vi "fgv_params_save-load_manual.vi"(7 "cmd":T8(ring), 8 "error in":errorcluster, 11 "file name":string) -> (0 "error out":errorcluster, 2 "Params_all":T1={"DL950_config"={"Timeout"=10000, "Time Div"=19, "Acq Mode"=0, "Record Len"=5, "Record Num"=0, "Start Point"=0, "End Poin"=60000, "Visa"="TCPIP0::192.168.0.100::inst0::INSTR", "Config Voltage"=[{"Enable"=TRUE, "Ch"=0, "V Div"=12, "Coupling"=1, "Probe"=3, "Act.Items"=FALSE, "items"=[]}, {"Enable"=TRUE, "Ch"=0, "V Div"=12, "Coupling"=1, "Probe"=3, "Act.Items"=FALSE, "items"=[]}], "Trigger on"=FALSE, "Trigger Level"=0.0, "Reset"=FALSE, "Config Temp"=[], "Trig Mode"=1, "Trig Pos"=50.0, "Trigger Slope"=0, "Trigger Source "=1, "Trig Start -5"=-5.0, "End 5"=5.0}, "BP4610 Config"={"VISA"="", "Limit-BP"={"Set"=enum."Current", "Voltage+[V]"=20.0, "Current+[A]"=5.0, "Voltage-[V]"=-20.0, "Current-[A]"=-5.0}, "SET BP"={"Set"=enum."FREQ/WAVE", "Operation mode"=0, "Voltage[Vp-p]"=0.0, "Current[Ap-p]"=0.0, "Voltage[V]"=0.0, "Current[A]"=0.0, "Frequency[Hz]"=1.0, "Waveform"=enum."Sine"}}, "DSP1950 Config"={"Port"="TCPIP0::192.168.0.14::HISLIP0::INSTR", "OVP Level"=0.0, "OCP Level"=0.0, "Current"=0.0, "Voltage"=0.0}, "DMM 2470 Config"={"Source Mode"=enum."Voltage", "Source Limit Level"=0.01, "Source Level"=0.0, "Output_2470"=FALSE}, "cDAQ-9221 Config"={"input terminal"=10083, "minimum value"=-60.0, "maximum value"=60.0, "number of samples"=1000, "rate"=10000.0, "sample mode"=10123, "physical channels"=""}, "cDAQ-9467 Config"="", "cDAQ-9269 AO Config"={"Ch"="cDAQ1Mod1/ao0", "Max V"=5.0, "Min V"=-5.0, " Rate"=1000.0, "N pts"=100, "sample mode"=10178}, "AO_Wave-config"={"offset"=0.0, "Samples"=0, "duty"=0.0, "Rate"=0.0, "wfm"={"Freq"=0.0, "Amp"=0.0, "Type"=enum."Sine Wave"}}, "DSP1950 Config LV"={"Port"="TCPIP0::192.168.0.14::HISLIP0::INSTR", "OVP Level"=0.0, "OCP Level"=0.0, "Current"=0.0, "Voltage"=0.0}} {"DSP1950 Config LV"."OCP Level" format="%#_13g"; "DSP1950 Config LV"."OVP Level" format="%#_13g"; "cDAQ-9269 AO Config"."sample mode" items=["유한 샘플"=10178, "연속 샘플"=10123, "하드웨어 타이밍에 의한 단일 포인트"=12522]; "cDAQ-9221 Config"."sample mode" items=["Finite Samples"=10178, "Continuous Samples"=10123, "Hardware Timed Single Point"=12522]; "cDAQ-9221 Config"."rate" format="%0.2f"; "cDAQ-9221 Config"."maximum value" format="%^.2e"; "cDAQ-9221 Config"."minimum value" format="%^.2e"; "cDAQ-9221 Config"."input terminal" items=["default"=-1, "RSE"=10083, "NRSE"=10078, "Differential"=10106, "Pseudodifferential"=12529]; "DSP1950 Config"."OCP Level" format="%#_13g"; "DSP1950 Config"."OVP Level" format="%#_13g"; "BP4610 Config"."SET BP"."Frequency[Hz]" min=1.0 max=100000.0 step=0.1; "BP4610 Config"."SET BP"."Current[A]" min=-20.0 max=20.0 step=0.001; "BP4610 Config"."SET BP"."Voltage[V]" min=-115.0 max=115.0 step=0.01; "BP4610 Config"."SET BP"."Current[Ap-p]" min=0.0 max=60.0 step=0.01; "BP4610 Config"."SET BP"."Voltage[Vp-p]" min=0.0 max=120.0 step=0.1; "BP4610 Config"."SET BP"."Operation mode" items=["CV-INT", "CV-EXT", "CV-ADD", "CC-INT", "CC-EXT", "CC-ADD"]; "BP4610 Config"."Limit-BP"."Current-[A]" min=-20.0 max=20.0 step=0.001; "BP4610 Config"."Limit-BP"."Voltage-[V]" min=-115.0 max=115.0 step=0.01; "BP4610 Config"."Limit-BP"."Current+[A]" min=0.0 max=60.0 step=0.01; "BP4610 Config"."Limit-BP"."Voltage+[V]" min=0.0 max=120.0 step=0.1; "DL950_config"."End 5" format="%.2g"; "DL950_config"."Trig Start -5" format="%.2f"; "DL950_config"."Trigger Source" items=["", "CH1", "CH2", "CH3", "CH4", "CH5", "CH6", "CH7", "CH8", "CH9", "CH10", "CH11", "CH12", "CH13", "CH14", "CH15", "CH16", "RMATH1", "RMATH2", "RMATH3", "RMATH4", "RMATH5", "RMATH6", "RMATH7", "RMATH8", "RMATH9", "RMATH10", "RMATH11", "RMATH12", "RMATH13", "RMATH14", "RMATH15", "RMATH16"]; "DL950_config"."Trigger Slope" items=["Rising", "Falling", "Both"]; "DL950_config"."Trig Pos" format="%.1f"; "DL950_config"."Trig Mode" items=["Normal", "Auto", "Auto Level", "Single", "Single(N)", "On Start", "No Set"]; "DL950_config"."Config Temp"."Type" items=["K", "E", "J", "T", "L", "U", "N", "R", "S", "B", "W", "Au7fe"]; "DL950_config"."Config Temp"."Channel" items=["", "CH1", "CH2", "CH3", "CH4", "CH5", "CH6", "CH7", "CH8", "CH9", "CH10", "CH11", "CH12", "CH13", "CH14", "CH15", "CH16"]; "DL950_config"."Trigger Level" format="%.3p"; "DL950_config"."Config Voltage"."items" items=["Peak to Peak", "Amplitude", "Max", "Min", "High", "Low", "Average", "Middle", "Rms", "Standard Deviation", "+Overshoot", "-Overshoot", "Rise", "Fall", "Frequency", "Period", "+Width", "-Width", "Duty Cycle", "Pulse Count", "Burst1 Width", "Burst2 Width", "Average Frequency", "Average Period", "Int1TY", "Int2TY"]; "DL950_config"."Config Voltage"."Probe" items=["1:1", "2:1", "5:1", "10:1", "20:1", "50:1", "100:1", "200:1", "500:1", "1000:1", "2000:1", "5000:1", "10k:1", "20k:1", "50k:1", "0.1A:1V", "0.2A:1V", "0.5A:1V", "1A:1V", "2A:1V", "5A:1V", "10A:1V", "20A:1V", "50A:1V", "100A:1V", "200A:1V", "250A:1V", "400A:1V", "500A:1V", "1kA:1V", "2kA:1V", "5kA:1V", "10kA:1V", "20kA:1V", "50kA:1V", "NoSet"]; "DL950_config"."Config Voltage"."Ch" items=["None", "CH1", "CH2", "CH3", "CH4", "CH5", "CH6", "CH7", "CH8", "CH9", "CH10", "CH11", "CH12", "CH13", "CH14", "CH15", "CH16", "MATH1", "MATH2", "MATH3", "MATH4", "MATH5", "MATH6", "MATH7", "MATH8", "EVENT"]; "DL950_config"."Config Voltage"."Coupling" items=["AC", "DC", "Ground", "AC-RMS", "DC-RMS"]; "DL950_config"."Config Voltage"."V Div" items=["0.1m", "0.2m", "0.5m", "1m", "2m", "5m", "10m", "20m", "50m", "100m", "200m", "500m", "1", "2", "4", "5", "8", "10", "20", "40", "50", "80", "100", "200", "400", "500", "800", "1k", "2k", "4k", "5k", "8k", "10k", "20k", "25k", "50k", "100k", "250k", "500k", "1000k"]; "DL950_config"."Record Len" items=["10k", "25k", "50k", "100k", "250k", "500k", "1M", "2.5M", "5M", "10M", "25M", "50M", "100M", "250M", "500M", "1G", "2G", "4G", "5G", "10G", "20G", "50G"]; "DL950_config"."Acq Mode" items=["Normal", "Average", "Envelope"]; "DL950_config"."Time Div" items=["100ns", "200ns", "500ns", "1us", "2us", "5us", "10us", "20us", "50us", "100us", "200us", "500us", "1ms", "2ms", "5ms", "10ms", "20ms", "50ms", "100ms", "200ms", "500ms", "1s", "2s", "3s", "4s", "5s", "6s", "10s", "20s", "30s", "1min", "2min", "3min", "4min", "5min", "6min", "10min", "12min", "30min", "1hour", "2hour", "3hour", "4hour", "5hour", "6hour", "8hour", "10hour", "12hour", "1day", "2day", "3day", "4day", "5day"]}, 3 "open cancelled":bool caption="취소됨")   [LabVIEW 2019]
uses:
  Tpye_ParaAll.ctl
  _ctrl/DL950_config.ctl
  _ctrl/BP4610_config.ctl
  _ctrl/DSP_config.ctl
  Devices/NI Board/cDAQ-9221 AI/Set_NIAI.ctl
  _ctrl/cDAQ-9269 Config.ctl
  Devices/NI Board/cDAQ-9269 AO/Set_AO_Wave-config.ctl
  Global_params.vi
  <vilib>/Utility/xml.llb/Write to XML File(string).vi
  <vilib>/Utility/xml.llb/Read From XML File(string).vi
panel:
  # "C 전압1"
  # "C 전압2"
  # "출력전압(+)"
  # "출력전압(-)"
  # "입력전류"
  # "출력전류"
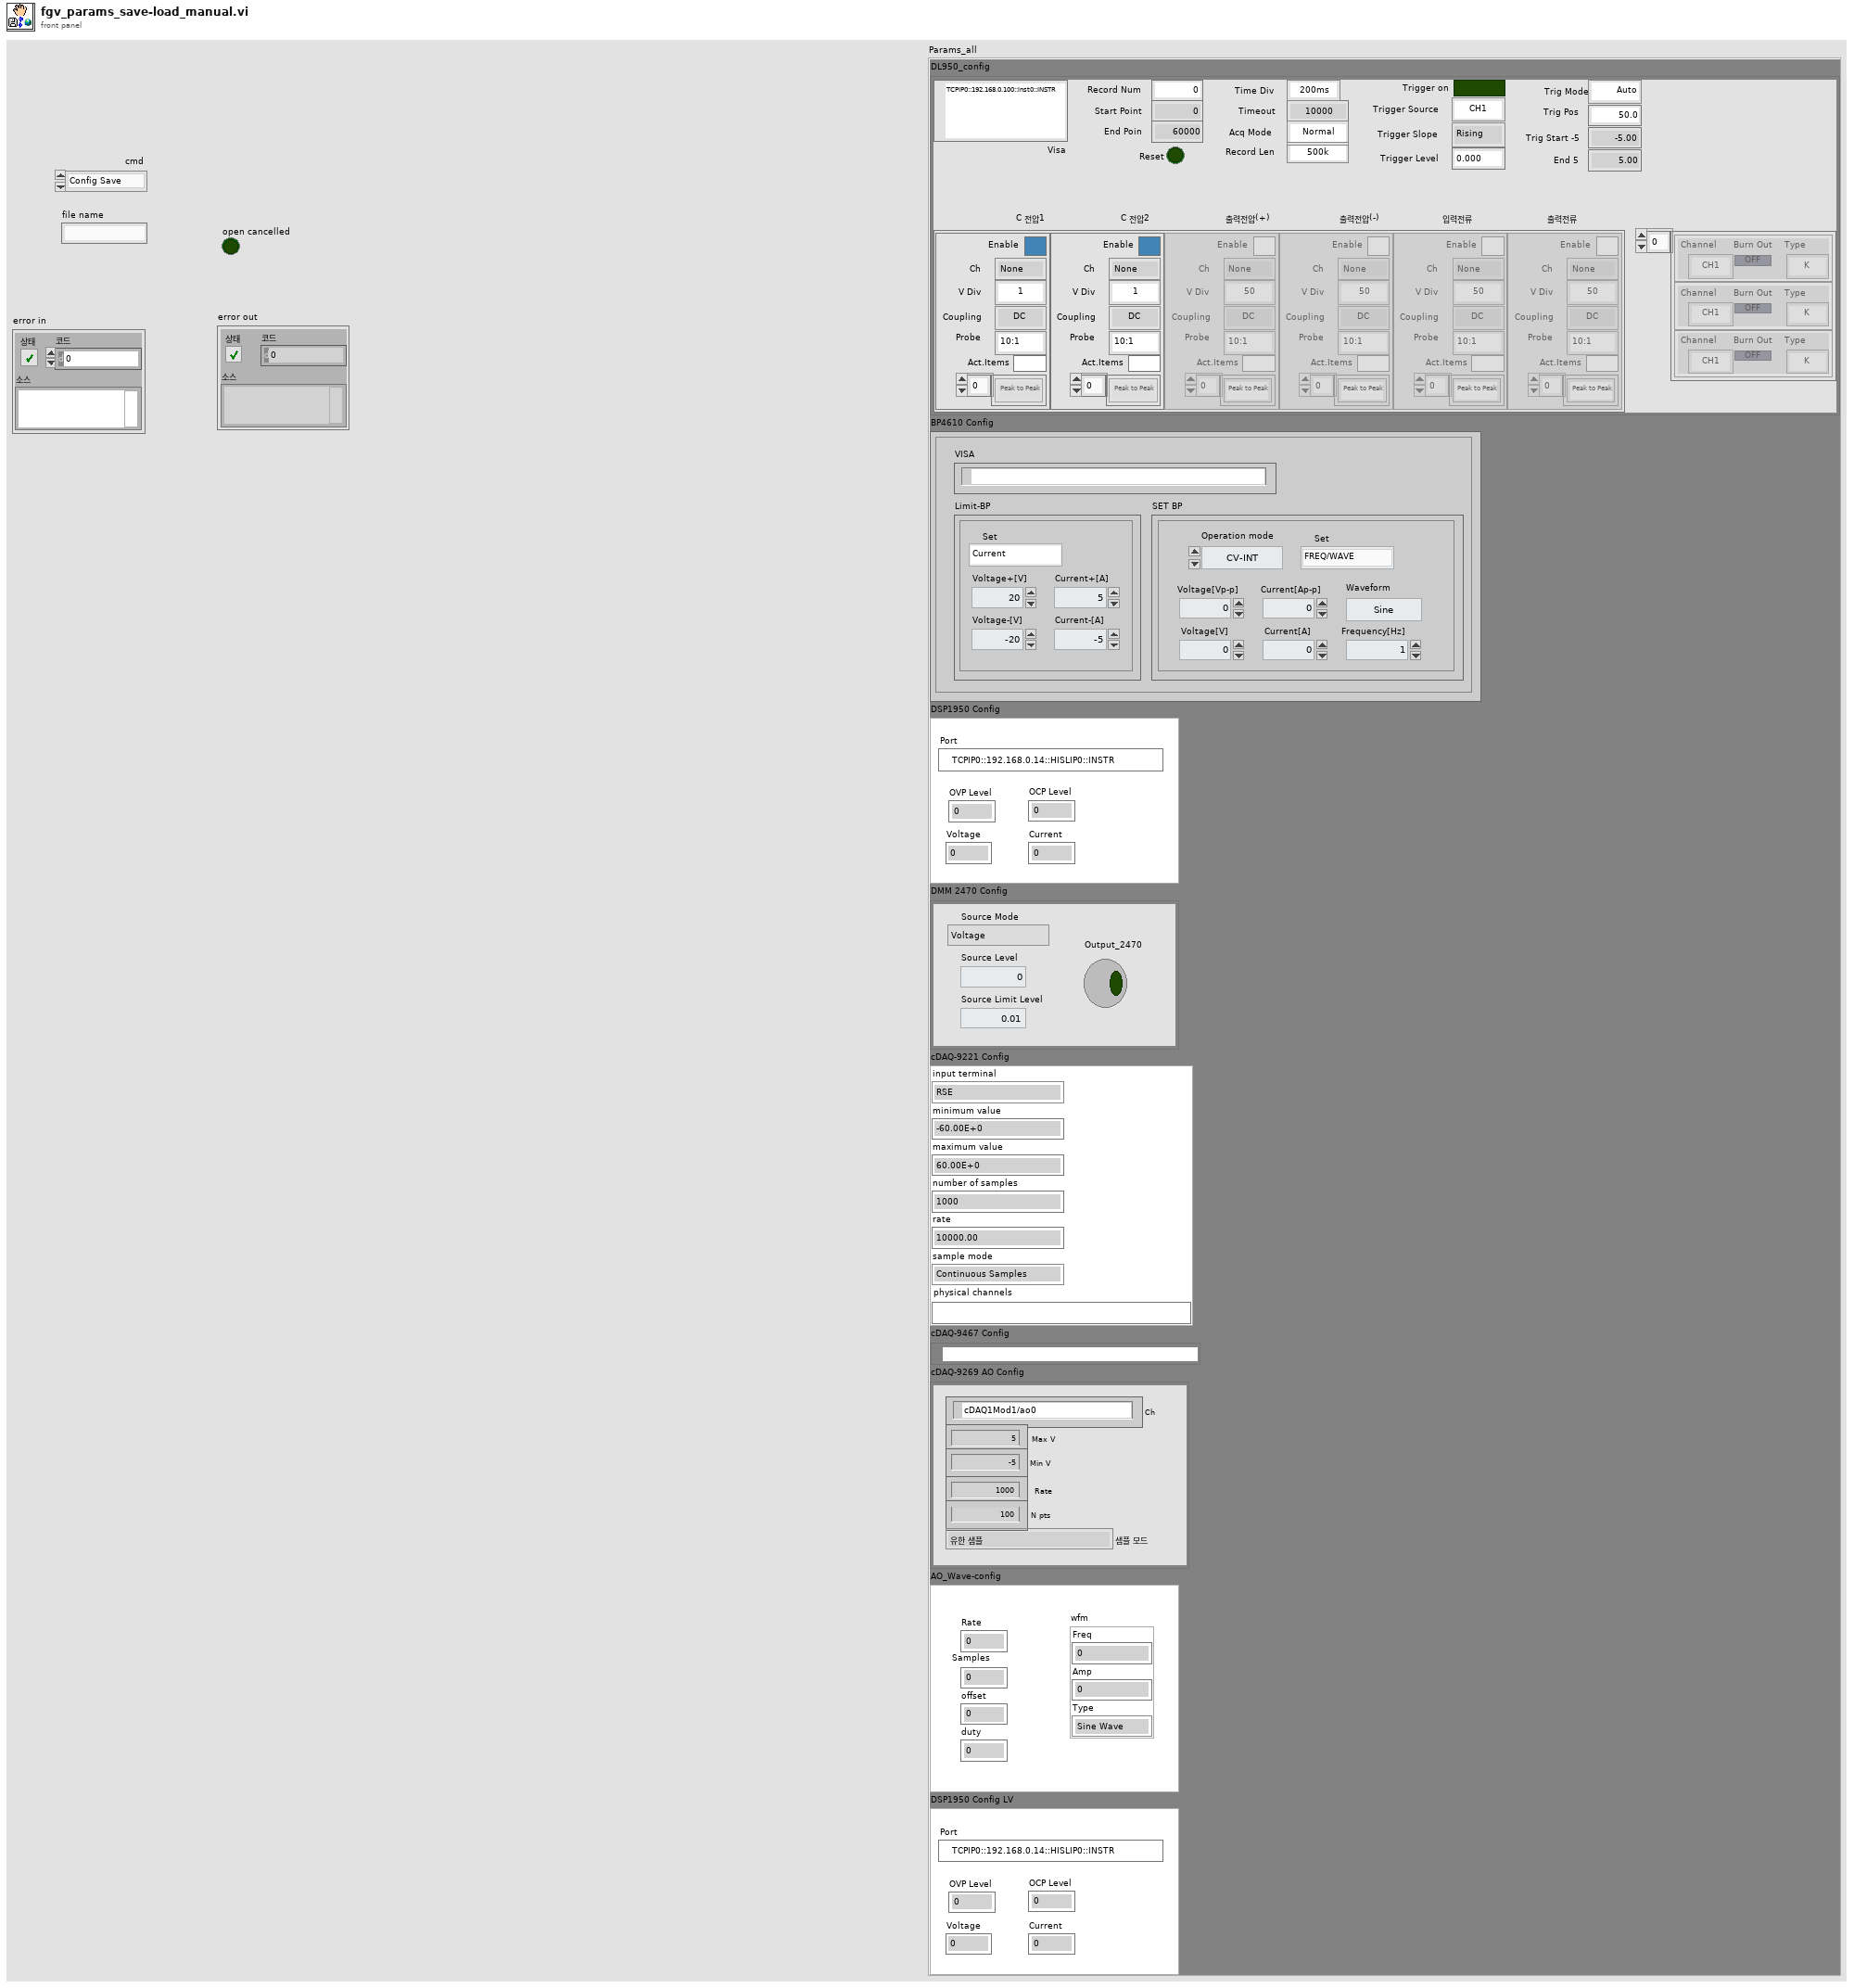
[diagram p1: front panel]
types:
  T1 = typedef "Tpye_ParaAll.ctl" = cluster{"DL950_config":T2, "BP4610 Config":T3, "DSP1950 Config":T4, "DMM 2470 Config":cluster{"Source Mode":enum16{"Voltage", "Current"}, "Source Limit Level":dbl, "Source Level":dbl, "Output_2470":bool}, "cDAQ-9221 Config":T5, "cDAQ-9467 Config":tag, "cDAQ-9269 AO Config":T6, "AO_Wave-config":T7, "DSP1950 Config LV":T4}
  T2 = typedef "DL950_config.ctl" = cluster{"Timeout":u32, "Time Div":i32, "Acq Mode":i32, "Record Len":i32, "Record Num":i32, "Start Point":i64, "End Poin":i64, "Visa":refnum<visa-resource-name>, "Config Voltage":cluster{"Enable":bool, "Ch":u16, "V Div":i32, "Coupling":i32, "Probe":i32, "Act.Items":bool, "items":i32[]}[], "Trigger on":bool, "Trigger Level":dbl, "Reset":bool, "Config Temp":cluster{"Channel":u16, "Burn Out":bool, " Type ":i32}[], "Trig Mode":i32, "Trig Pos":dbl, "Trigger Slope":i32, "Trigger Source ":i32, "Trig Start -5":dbl, "End 5":dbl}
  T3 = typedef "BP4610_config.ctl" = cluster{"VISA":refnum<visa-resource-name>, "Limit-BP":cluster{"Set":enum16{"Current", "Voltage"}, "Voltage+[V]":dbl, "Current+[A]":dbl, "Voltage-[V]":dbl, "Current-[A]":dbl}, "SET BP":cluster{"Set":enum16{"Current", "Voltage", "FREQ/WAVE"}, "Operation mode":u16, "Voltage[Vp-p]":dbl, "Current[Ap-p]":dbl, "Voltage[V]":dbl, "Current[A]":dbl, "Frequency[Hz]":dbl, "Waveform":enum16{"Sine", "Square", "ARB 1", "ARB 2", "ARB 3", "ARB 4", "ARB 5", "ARB 6", "ARB 7", "ARB 8", "ARB 9", "ARB 10", "ARB 11", "ARB 12", "ARB 13", "ARB 14", "ARB 15", "ARB 16"}}}
  T4 = typedef "DSP_config.ctl" = cluster{"Port":refnum<visa-resource-name>, "OVP Level":dbl, "OCP Level":dbl, "Current":dbl, "Voltage":dbl}
  T5 = typedef "Set_NIAI.ctl" = cluster{"input terminal":i32, "minimum value":dbl, "maximum value":dbl, "number of samples":i32, "rate":dbl, "sample mode":i32, "physical channels":tag}
  T6 = typedef "cDAQ-9269 Config.ctl" = cluster{"Ch":tag, "Max V":dbl, "Min V":dbl, " Rate":dbl, "N pts":i32, "sample mode":i32}
  T7 = typedef "Set_AO_Wave-config.ctl" = cluster{"offset":dbl, "Samples":i32, "duty":dbl, "Rate":dbl, "wfm":cluster{"Freq":dbl, "Amp":dbl, "Type":enum16{"Sine Wave", "Triangle Wave", "Square Wave", "Sawtooth Wave"}}}
  T8 = enum16{"Config Save", "Config Load", "LastRUN Save", "LastRUN Load"}
  T9 = enum16{"open", "replace", "create", "open or create", "replace or create", "replace or create with confirmation"}
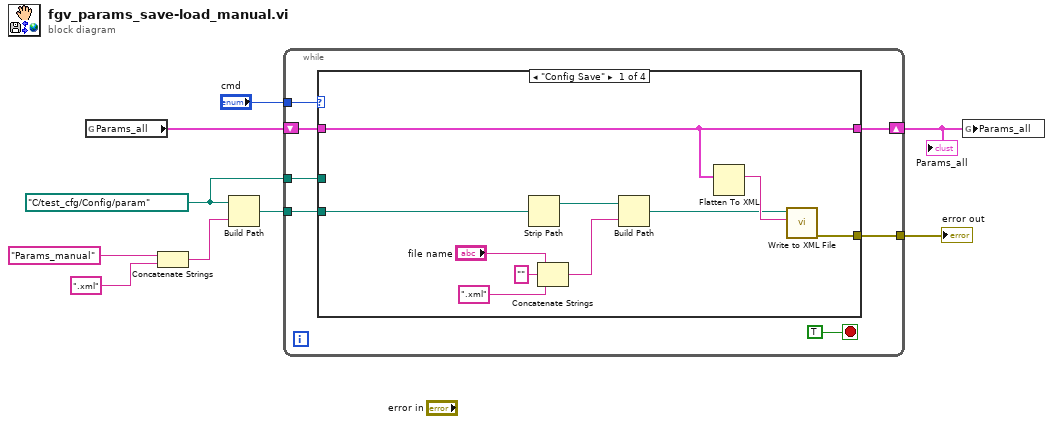
[diagram p0: block diagram]
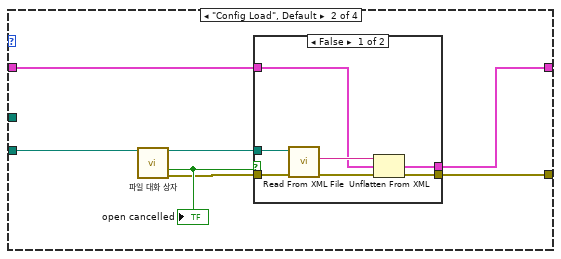
[diagram p2: hidden frame]
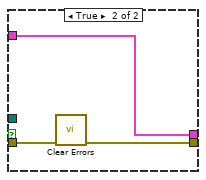
[diagram p3: hidden frame]
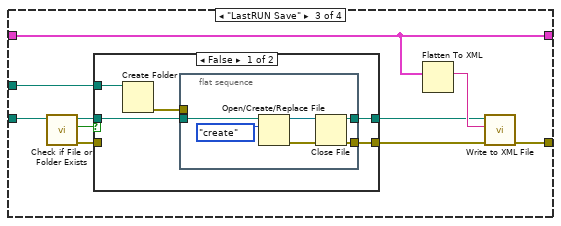
[diagram p4: hidden frame]
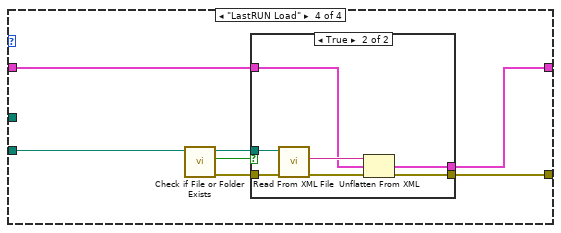
[diagram p6: hidden frame]
diagram:
  w8 = path "C:/test_cfg/Config/param" ("XML File Path")
  n1 = global read "Global_params.vi" "Params_all"() -> (w2:T1)
  n2 = Concatenate Strings("Params_manual" ("string"), ".xml" ("string")) -> (w4:string)
  n3 = Build Path(base path=w8, name or relative path=w4) -> (appended path=w9:path)
  n4 = while {
    tunnel: [w16] -> w7
    tunnel: "cmd" -> [w15]
    tunnel: w9 -> [w13]
    shift-right: [w12] -> w1
    shift-left: w2 -> [w14]
    tunnel: w8 -> [w10]
    stop <- TRUE stop-if-true
    n5 = case shown="\"Config Save\"" w15 {
      tunnel: w14 -> [w21 w30 w47 w73]
      tunnel: w13 -> [w24 w33 w46 w67]
      tunnel: [w25 w28 w48 w71] -> w16
      tunnel: [w21 w27 w47 w72] -> w12
      tunnel: w10 -> [_ _ w44 _]
      frame "Config Save" {
        n6 = Strip Path(path=w24) -> (stripped path=w23:path)  [unwired: 1 out]
        n7 = Concatenate Strings("file name", "" ("문자열"), ".xml" ("문자열")) -> (w22:string)
        n8 = Build Path(base path=w23, name or relative path=w22) -> (appended path=w18:path)
        n9 = Flatten To XML(anything=w21) -> (xml string=w26:string)
        n10 = call-poly <vilib>:"Write to XML File.vi"("XML Input"=w26, "XML File Path"=w18) -> ("error out"=w25:errorcluster)  [unwired: 7 in, 2 out]
      }
      frame "Config Load", Default {
        n11 = call "파일 대화 상자"("start path"=w33) -> ("selected path"=w31:path, "cancelled"=w32:bool, "error out"=w29:errorcluster)  [unwired: 11 in, 1 out]
        "open cancelled" <- w32
        n12 = case shown="False" w32 {
          tunnel: w31 -> [w39 _]
          tunnel: w30 -> [w38 w43]
          tunnel: [w37 w43] -> w27
          tunnel: w29 -> [w35 w42]
          tunnel: [w34 w41] -> w28
          frame False {
            n13 = call-poly <vilib>:"Read From XML File.vi"("error in (no error)"=w35, "XML File Path"=w39) -> ("error out"=w36:errorcluster, "XML Elements"=w40:string)  [unwired: 7 in, 1 out]
            n14 = Unflatten From XML(xml string=w40, type=w38, error in (no error)=w36) -> (value=w37:T1, error out=w34:errorcluster)
          }
          frame True {
            n15 = call <vilib>:"Clear Errors.vi"("error in (no error)"=w42) -> ("error out"=w41:errorcluster)  [unwired: 5 in, 1 out]
          }
        }
      }
      frame "LastRUN Save" {
        n16 = call <vilib>:"Check if File or Folder Exists.vi"("path"=w46) -> ("error out"=w52:errorcluster, "file or folder exists?"=w50:bool, "dup path"=w51:path)  [unwired: 8 in]
        n17 = case shown="False" w50 {
          tunnel: w52 -> [_ w66]
          tunnel: w51 -> [w58 w65]
          tunnel: [w56 w66] -> w49
          tunnel: [w57 w65] -> w45
          tunnel: w44 -> [w55 _]
          frame False {
            n18 = Create Folder(path (use dialog)=w55) -> (error out=w54:errorcluster)  [unwired: 2 in, 2 out]
            n19 = flat-sequence {
              tunnel: w58 -> [w64]
              tunnel: [w60] -> w57
              tunnel: [w59] -> w56
              tunnel: w54 -> [_]
              frame #0 {
                n20 = Open/Create/Replace File(file path (use dialog)=w64, operation (0:open)=T9."create" ("동작(0:open)")) -> (refnum out=w61:refnum<file>, error out=w62:errorcluster)  [unwired: 4 in, 1 out]
                n21 = Close File(refnum=w61, error in=w62) -> (path=w60:path, error out=w59:errorcluster)
              }
            }
          }
          frame True {
          }
        }
        n22 = Flatten To XML(anything=w47) -> (xml string=w53:string)
        n23 = call-poly <vilib>:"Write to XML File.vi"("error in (no error)"=w49, "XML Input"=w53, "XML File Path"=w45) -> ("error out"=w48:errorcluster)  [unwired: 6 in, 2 out]
      }
      frame "LastRUN Load" {
        n24 = call <vilib>:"Check if File or Folder Exists.vi"("path"=w67) -> ("error out"=w68:errorcluster, "file or folder exists?"=w69:bool, "dup path"=w70:path)  [unwired: 8 in]
        n25 = case shown="True" w69 {
          tunnel: w73 -> [_ w80]
          tunnel: [_ w79] -> w72
          tunnel: [w74 w77] -> w71
          tunnel: w70 -> [_ w76]
          tunnel: w68 -> [w74 w75]
          frame False {
          }
          frame True {
            n26 = call-poly <vilib>:"Read From XML File.vi"("error in (no error)"=w75, "XML File Path"=w76) -> ("error out"=w78:errorcluster, "XML Elements"=w81:string)  [unwired: 7 in, 1 out]
            n27 = Unflatten From XML(xml string=w81, type=w80, error in (no error)=w78) -> (value=w79:T1, error out=w77:errorcluster)
          }
        }
      }
    }
  }
  "error out" <- w7
  "Params_all" <- w1
  n28 = global write "Global_params.vi" "Params_all"(w1) -> ()
